vi "GetActualDriveDistance.vi"(8 "Robot Motion Commands In":T1, 9 "Zero Encoder":bool) -> (3 "Robot Motion Commands Out":T1)   [LabVIEW 2018]
uses:
  Controls/Robot Pivot Motion Commands.ctl
  Controls/Pivot Motor Commands.ctl
  Controls/Robot Drive Mode.ctl
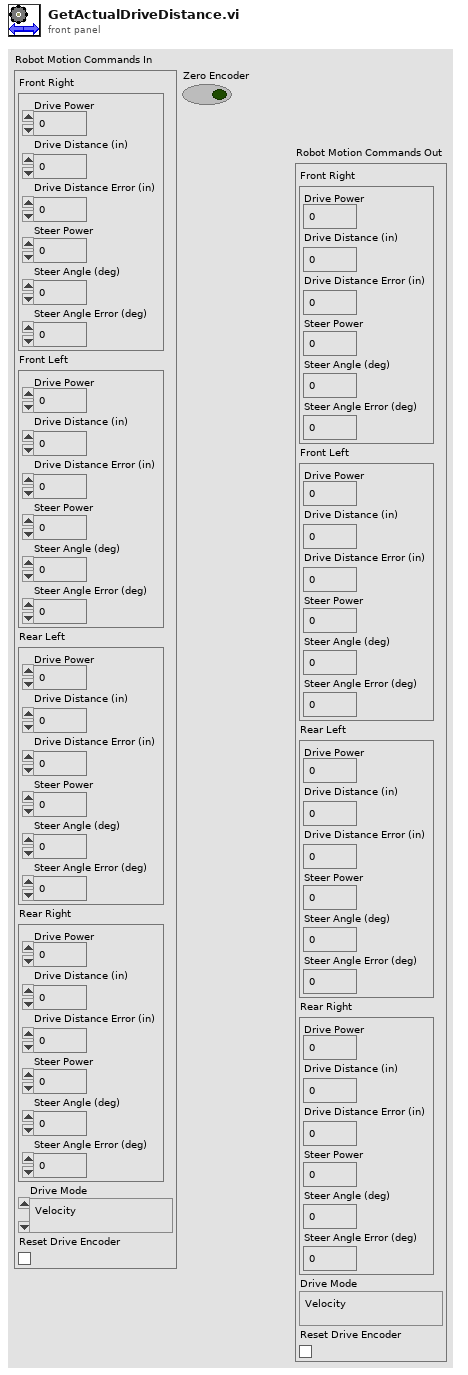
[diagram p1: front panel]
types:
  T1 = typedef "Robot Pivot Motion Commands.ctl" = cluster{"Front Right":T2, "Front Left":T2, "Rear Left":T2, "Rear Right":T2, "Drive Mode":T3, "Reset Drive Encoder":bool}
  T2 = typedef "Pivot Motor Commands.ctl" = cluster{"Drive Power":dbl, "Drive Distance (in)":dbl, "Drive Distance Error (in)":dbl, "Steer Power":dbl, "Steer Angle (deg)":dbl, "Steer Angle Error (deg)":dbl}
  T3 = typedef "Robot Drive Mode.ctl" = enum16{"Velocity", "Distance"}
  T4 = typedef "WPI_EncoderDevRef.ctl" = cluster{"DevStatus":errorcluster, "EncoderIndex":T5, "CounterIndex":T6, "DistancePerCount":dbl, "Decoding Type":T7}
  T5 = typedef "FPGA_EncoderIdx.ctl" = enum8{"Enc 0", "Enc 1", "Enc 2", "Enc 3", "Enc 4", "Enc 5", "Enc 6", "Enc 7", "Invalid"}
  T6 = typedef "FPGA_CounterCtrSystemIndex.ctl" = enum8{"Ctr 0", "Ctr 1", "Ctr 2", "Ctr 3", "Ctr 4", "Ctr 5", "Ctr 6", "Ctr 7", "Invalid"}
  T7 = typedef "WPI_EncoderType.ctl" = enum16{"1x", "2x", "4x"}
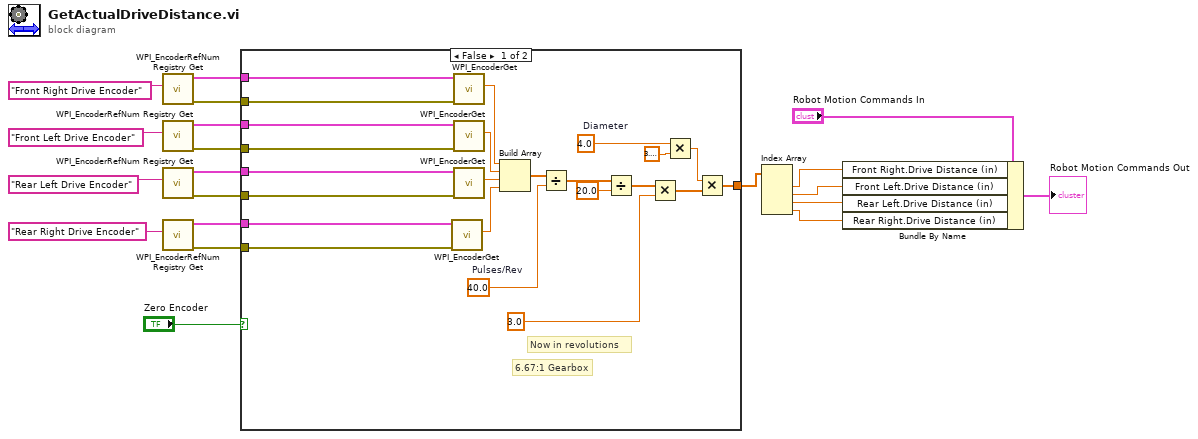
[diagram p0: block diagram]
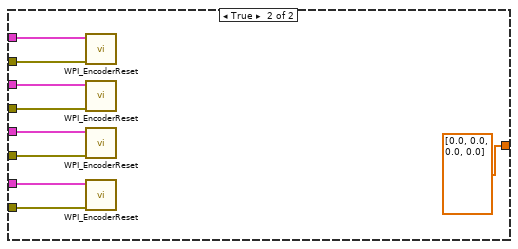
[diagram p2: hidden frame]
diagram:
  n1 = call <vilib>:"WPI_EncoderRefNum Registry Get.vi"("refnum name"="Front Right Drive Encoder") -> ("error out"=w3:errorcluster, "EncoderDevRef"=w2:T4)  [unwired: 9 in]
  n2 = call <vilib>:"WPI_EncoderRefNum Registry Get.vi"("refnum name"="Front Left Drive Encoder") -> ("error out"=w5:errorcluster, "EncoderDevRef"=w4:T4)  [unwired: 9 in]
  n3 = call <vilib>:"WPI_EncoderRefNum Registry Get.vi"("refnum name"="Rear Left Drive Encoder") -> ("error out"=w7:errorcluster, "EncoderDevRef"=w6:T4)  [unwired: 9 in]
  n4 = call <vilib>:"WPI_EncoderRefNum Registry Get.vi"("refnum name"="Rear Right Drive Encoder") -> ("error out"=w9:errorcluster, "EncoderDevRef"=w8:T4)  [unwired: 9 in]
  n5 = case shown="False" "Zero Encoder" {
    tunnel: [w29 dbl[] [0.0, 0.0, 0.0, 0.0]] -> w18
    tunnel: w9 -> [w28 w44]
    tunnel: w8 -> [w27 w45]
    tunnel: w7 -> [w26 w46]
    tunnel: w6 -> [w25 w47]
    tunnel: w5 -> [w24 w48]
    tunnel: w4 -> [w23 w49]
    tunnel: w3 -> [w22 w50]
    tunnel: w2 -> [w21 w51]
    frame False {
      w40 = 4.0  # Diameter
      w43 = 40.0  # Pulses/Rev
      # "Now in revolutions"
      # "6.67:1 Gearbox"
      n6 = call <vilib>:"WPI_EncoderGet.vi"("error in (no error)"=w28, "EncoderDevRef"=w27) -> ("Distance"=w31:dbl)  [unwired: 4 in, 5 out]
      n7 = call <vilib>:"WPI_EncoderGet.vi"("error in (no error)"=w22, "EncoderDevRef"=w21) -> ("Distance"=w34:dbl)  [unwired: 4 in, 5 out]
      n8 = call <vilib>:"WPI_EncoderGet.vi"("error in (no error)"=w24, "EncoderDevRef"=w23) -> ("Distance"=w33:dbl)  [unwired: 4 in, 5 out]
      n9 = call <vilib>:"WPI_EncoderGet.vi"("error in (no error)"=w26, "EncoderDevRef"=w25) -> ("Distance"=w32:dbl)  [unwired: 4 in, 5 out]
      n10 = Build Array(w34, w33, w32, w31) -> (w30:dbl[])
      n11 = Divide(x=w30, y=w43) -> (x/y=w42:dbl[])
      n12 = Divide(x=w42, y=20.0) -> (x/y=w37:dbl[])
      n13 = Multiply(x=w37, y=3.0) -> (x*y=w36:dbl[])
      n14 = Multiply(x=w40, y=3.141592653589793) -> (x*y=w38:dbl)
      n15 = Multiply(x=w38, y=w36) -> (x*y=w29:dbl[])
    }
    frame True {
      n16 = call <vilib>:"WPI_EncoderReset.vi"("error in (no error)"=w50, "EncoderDevRef"=w51) -> ()  [unwired: 8 in, 2 out]
      n17 = call <vilib>:"WPI_EncoderReset.vi"("error in (no error)"=w48, "EncoderDevRef"=w49) -> ()  [unwired: 8 in, 2 out]
      n18 = call <vilib>:"WPI_EncoderReset.vi"("error in (no error)"=w46, "EncoderDevRef"=w47) -> ()  [unwired: 8 in, 2 out]
      n19 = call <vilib>:"WPI_EncoderReset.vi"("error in (no error)"=w44, "EncoderDevRef"=w45) -> ()  [unwired: 8 in, 2 out]
    }
  }
  n20 = Index Array(array=w18) -> (element #1=w17:dbl, element #2=w16:dbl, element #3=w15:dbl, element #4=w14:dbl)  [unwired: 4 in]
  n21 = Bundle By Name(cluster="Robot Motion Commands In", "Front Right.Drive Distance (in)"=w17, "Front Left.Drive Distance (in)"=w16, "Rear Left.Drive Distance (in)"=w15, "Rear Right.Drive Distance (in)"=w14) -> (→"Robot Motion Commands Out":T1)
